vi "Servo.vi"(7 "Action":T1, 8 "error in (no error)":errorcluster, 10 "Angle (deg)":i32, 11 "ServoDeviceRef":T2={"DeviceStatus"={"status"=FALSE, "code"=0, "source"=""}, "Digital Module"=enum."Digital Module 1", "PWM Channel"=enum."Invalid", "DeadBand"={"Name"="", "maxPositivePwm"=0, "minPositivePwm"=0, "centerPwm"=0, "maxNegativePwm"=0, "minNegativePwm"=0, "angularRange"=0}}) -> (0 "error out":errorcluster, 2 "Angle (deg)":i32)   [LabVIEW 2013]
uses:
  <vilib>/Rock Robotics/WPI/PWM/Servo/WPI_ServoDeviceRef.ctl
  <vilib>/Rock Robotics/SystemInterfaces/Typedef/FPGA_TypedefDigitalModule.ctl
  <vilib>/Rock Robotics/SystemInterfaces/DIO/FPGA_DIOPWMChannel.ctl
  <vilib>/Rock Robotics/WPI/PWM/WPI_PWMDeadband.ctl
  ServoAction.ctl
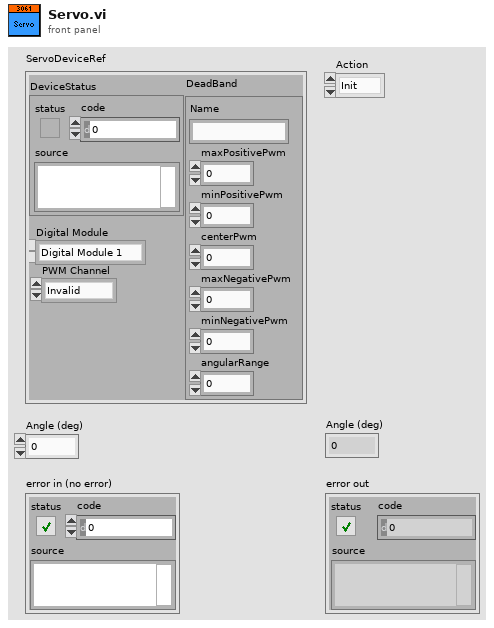
[diagram p1: front panel]
types:
  T1 = typedef "ServoAction.ctl" = enum16{"Init", "SetAngle", "GetAngle", "Lower", "Raise", "Disable"}
  T2 = typedef "WPI_ServoDeviceRef.ctl" = cluster{"DeviceStatus":errorcluster, "Digital Module":T3, "PWM Channel":T4, "DeadBand":T5}
  T3 = typedef "FPGA_TypedefDigitalModule.ctl" = enum16{"Digital Module 1", "Digital Module 2"}
  T4 = typedef "FPGA_DIOPWMChannel.ctl" = enum8{"PWM 1", "PWM 2", "PWM 3", "PWM 4", "PWM 5", "PWM 6", "PWM 7", "PWM 8", "PWM 9", "PWM 10", "Invalid"}
  T5 = typedef "WPI_PWMDeadband.ctl" = cluster{"Name":string, "maxPositivePwm":i32, "minPositivePwm":i32, "centerPwm":i32, "maxNegativePwm":i32, "minNegativePwm":i32, "angularRange":u16}
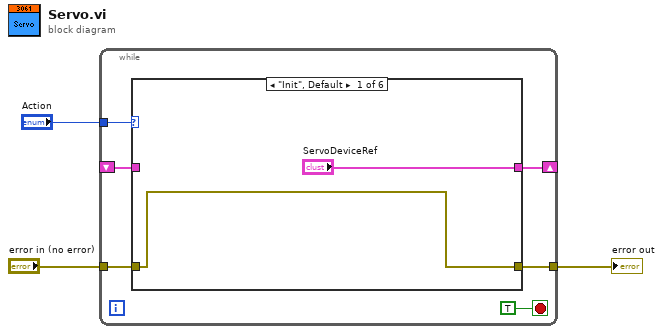
[diagram p0: block diagram]
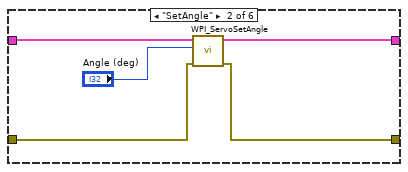
[diagram p2: hidden frame]
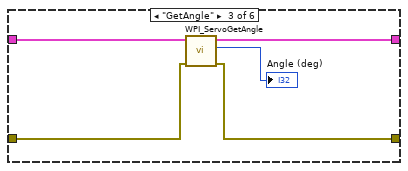
[diagram p3: hidden frame]
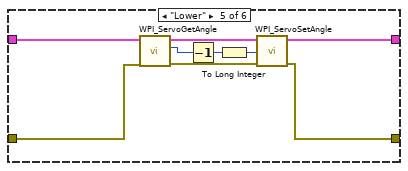
[diagram p5: hidden frame]
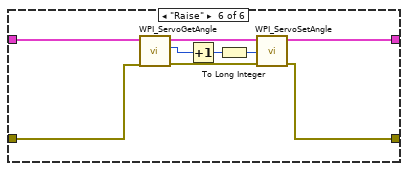
[diagram p6: hidden frame]
diagram:
  n1 = while {
    tunnel: "Action" -> [w8]
    shift-right: [w7] -> _
    shift-left: _ -> [w6]
    tunnel: "error in (no error)" -> [w5]
    tunnel: [w4] -> w1
    stop <- TRUE stop-if-true
    n2 = case shown="\"Init\", Default" w8 {
      tunnel: ["ServoDeviceRef" w14 w20 w22 w26 w39] -> w7
      tunnel: w6 -> [_ w15 w21 w22 w27 w41]
      tunnel: w5 -> [w10 w13 w19 w23 w25 w35]
      tunnel: [w10 w12 w18 w23 w24 w36] -> w4
      frame "Init", Default {
      }
      frame "SetAngle" {
        n3 = call <vilib>:"WPI_ServoSetAngle.vi"("error in (no error)"=w13, "Angle"="Angle (deg)", "ServoDeviceRef"=w15) -> ("error out"=w12:errorcluster, "ServoDeviceRef"=w14:T2)  [unwired: 7 in]
      }
      frame "GetAngle" {
        n4 = call <vilib>:"WPI_ServoGetAngle.vi"("ServoDeviceRef"=w21, "error in (no error)"=w19) -> ("ServoDeviceRef"=w20:T2, "Angle"=→"Angle (deg)":u16, "error out"=w18:errorcluster)  [unwired: 6 in]
      }
      frame "Disable" {
      }
      frame "Lower" {
        n5 = call <vilib>:"WPI_ServoGetAngle.vi"("ServoDeviceRef"=w27, "error in (no error)"=w25) -> ("ServoDeviceRef"=w32:T2, "Angle"=w31:u16, "error out"=w30:errorcluster)  [unwired: 6 in]
        n6 = Decrement(x=w31) -> (x-1=w29:u16)
        n7 = To Long Integer(number=w29) -> (32bit integer=w28:i32)
        n8 = call <vilib>:"WPI_ServoSetAngle.vi"("error in (no error)"=w30, "Angle"=w28, "ServoDeviceRef"=w32) -> ("error out"=w24:errorcluster, "ServoDeviceRef"=w26:T2)  [unwired: 7 in]
      }
      frame "Raise" {
        n9 = call <vilib>:"WPI_ServoGetAngle.vi"("ServoDeviceRef"=w41, "error in (no error)"=w35) -> ("ServoDeviceRef"=w40:T2, "Angle"=w38:u16, "error out"=w37:errorcluster)  [unwired: 6 in]
        n10 = Increment(x=w38) -> (x+1=w34:u16)
        n11 = To Long Integer(number=w34) -> (32bit integer=w33:i32)
        n12 = call <vilib>:"WPI_ServoSetAngle.vi"("error in (no error)"=w37, "Angle"=w33, "ServoDeviceRef"=w40) -> ("error out"=w36:errorcluster, "ServoDeviceRef"=w39:T2)  [unwired: 7 in]
      }
    }
  }
  "error out" <- w1
